vi "Read GPS Data.vi"(8 "error in (no error)":errorcluster, 11 "Simulator in":refnum<class "Simulator.lvclass">) -> (0 "error out":errorcluster, 2 "Current Location ( GPS )":cluster{"Latitude":dbl, "Longitude":dbl}, 3 "Simulator out":refnum<class "Simulator.lvclass">)   [LabVIEW 2011, in "Simulator.lvclass"]
uses:
  Simulator.lvclass
  Simulator.lvclass/Simulator.ctl
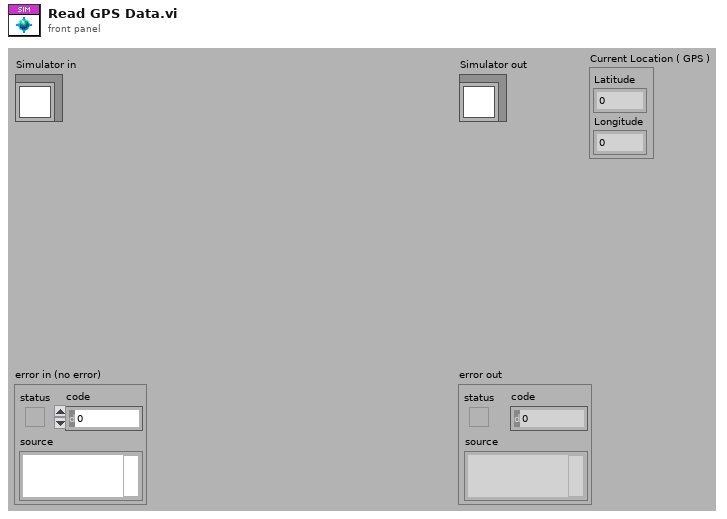
[diagram p1: front panel]
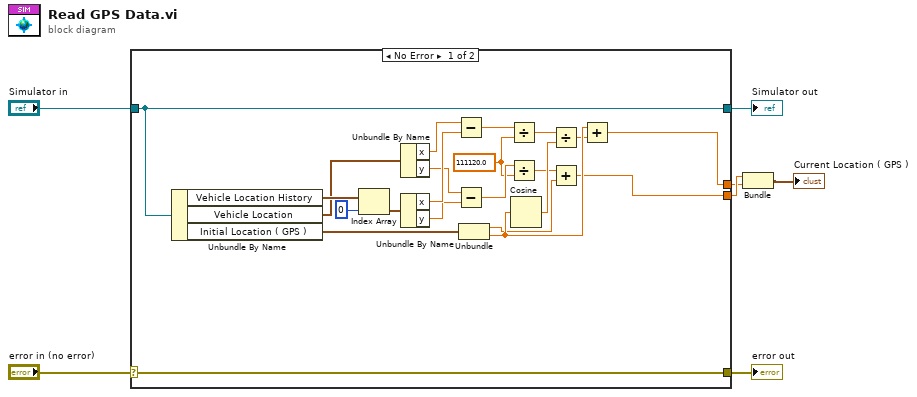
[diagram p0: block diagram]
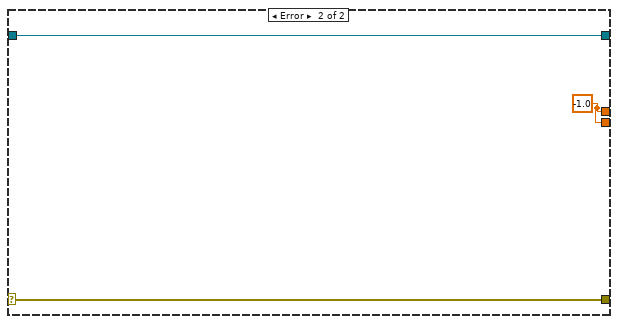
[diagram p2: hidden frame]
diagram:
  n1 = case shown="No Error" "error in (no error)" {
    selector: "error in (no error)" -> [w29 w32]
    tunnel: [w29 w32] -> w6
    tunnel: [w28 w31] -> w4
    tunnel: "Simulator in" -> [w28 w31]
    tunnel: [w13 w30] -> w2
    tunnel: [w12 w30] -> w1
    frame No Error {
      w20 = 111120.0 ("y")
      n2 = Unbundle By Name(w28) -> ("Vehicle Location History"=w27:cluster{"x":dbl, "y":dbl}[], "Vehicle Location"=w24:cluster{"x":dbl, "y":dbl}, "Initial Location ( GPS )"=w22:cluster{"Latitude":dbl, "Longitude":dbl})
      n3 = Index Array(array=w27, index=0) -> (element=w25:cluster{"x":dbl, "y":dbl})
      n4 = Unbundle By Name(w24) -> ("x"=w11:dbl, "y"=w8:dbl)
      n5 = Unbundle By Name(w25) -> ("x"=w10:dbl, "y"=w9:dbl)
      n6 = Subtract(x=w11, y=w10) -> (x-y=w21:dbl)
      n7 = Subtract(x=w8, y=w9) -> (x-y=w23:dbl)
      n8 = Unbundle(w22) -> ("Latitude"=w14:dbl, "Longitude"=w17:dbl)
      n9 = Divide(x=w21, y=w20) -> (x/y=w19:dbl)
      n10 = Divide(x=w23, y=w20) -> (x/y=w15:dbl)
      n11 = Cosine(x=w17) -> (cos(x)=w18:dbl)
      n12 = Divide(x=w19, y=w18) -> (x/y=w16:dbl)
      n13 = Add(x=w15, y=w14) -> (x+y=w13:dbl)
      n14 = Add(x=w17, y=w16) -> (x+y=w12:dbl)
    }
    frame Error {
      w30 = -1.0
    }
  }
  "error out" <- w6
  "Simulator out" <- w4
  n15 = Bundle(w2, w1) -> (→"Current Location ( GPS )":cluster{dbl, dbl})  [unwired: 1 in]
